vi "Shutdown.vi"(8 "error in":errorcluster, 11 "tCRD in":refnum<class "Open Path CRD.lvclass">) -> (0 "error out":errorcluster, 3 "tCRD out":refnum<class "Open Path CRD.lvclass">)   [LabVIEW 2015, in "Open Path CRD.lvclass"]
uses:
  Open Path CRD.lvclass
  Reusable/Session APIs/File Access/Base/File Session.lvclass
  Open Path CRD.lvclass/Open Path CRD.ctl
  <vilib>/FPGAPlugInAG/sbRIO-9637/niLvFpga_Close_sbRIO-9637.vi
  Reusable/CRDS/Main/CRDS.lvclass
  <vilib>/rvi/interface/nirviCloseFPGA/nirviCloseFPGA.xnode
  Open Path FPGA Ref.ctl
  FPGA Bitfiles/80MHz_server.lvbitx
  Devices/Alicat/Session Based/Alicat Device.lvclass
  Devices/CR5/CR5.lvclass
  <userlib>/_Session Fwk/Session - Root.lvclass
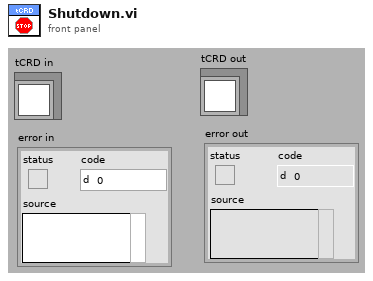
[diagram p1: front panel]
types:
  T1 = typedef "Open Path CRD.lvclass/Open Path FPGA Ref.ctl" = refnum<k20>
  T2 = typedef "Config Data.lvclass/Config Session.ctl" = refnum<data-value>
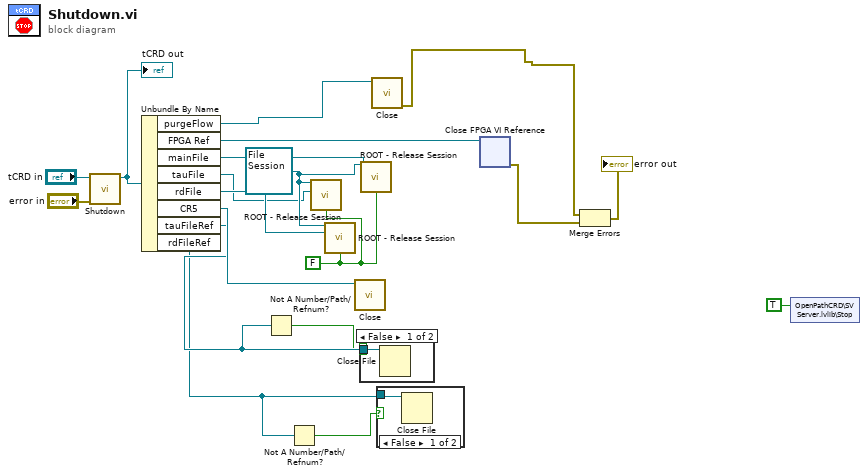
[diagram p0: block diagram]
diagram:
  w6 = FALSE ("force destroy? (F)")
  w10 = refnum<class "File Session.lvclass"> refnum ("File Session")
  n1 = call-parent "Shutdown.vi"("error in"="error in", "Instrument in"="tCRD in") -> ("Instrument out"=w17:refnum<class "Open Path CRD.lvclass">)  [unwired: 8 in, 1 out]
  "tCRD out" <- w17
  n2 = Unbundle By Name(w17) -> ("purgeFlow"=w13:refnum<class "Alicat Device.lvclass">, "FPGA Ref"=w16:T1, "mainFile"=w7:T2, "tauFile"=w8:T2, "rdFile"=w9:T2, "CR5"=w11:refnum<class "CR5.lvclass">, "tauFileRef"=w4:refnum<file>, "rdFileRef"=w3:refnum<file>)
  n3 = Not A Number/Path/Refnum?(number/path/refnum=w4) -> (NaN/Path/Refnum?=w1:bool)
  n4 = Not A Number/Path/Refnum?(number/path/refnum=w3) -> (NaN/Path/Refnum?=w2:bool)
  n5 = call <userlib>:"ROOT - Release Session.vi"("OBJ - Session in"=w10, "Session Handle in"=w8, "force destroy? (F)"=w6) -> ()  [unwired: 11 in, 2 out]
  n6 = call <userlib>:"ROOT - Release Session.vi"("OBJ - Session in"=w10, "Session Handle in"=w9, "force destroy? (F)"=w6) -> ()  [unwired: 11 in, 2 out]
  n7 = call-dynamic "Close.vi"("CR5 in"=w11) -> ()  [unwired: 9 in, 2 out]
  n8 = case shown="False" w1 {
    tunnel: w4 -> [w20 _]
    frame False {
      n9 = Close File(refnum=w20) -> ()  [unwired: 1 in, 2 out]
    }
    frame True {
    }
  }
  n10 = call <userlib>:"ROOT - Release Session.vi"("OBJ - Session in"=w10, "Session Handle in"=w7, "force destroy? (F)"=w6) -> ()  [unwired: 11 in, 2 out]
  n11 = call-dynamic "Close.vi"("Cfg Dev in"=w13) -> ("error out"=w12:errorcluster)  [unwired: 9 in, 1 out]
  n12 = case shown="False" w2 {
    tunnel: w3 -> [w21 _]
    frame False {
      n13 = Close File(refnum=w21) -> ()  [unwired: 1 in, 2 out]
    }
    frame True {
    }
  }
  n14 = xnode "Close FPGA VI Reference"("FPGA VI Reference In"=w16) -> ("error out"=w15:errorcluster)  [unwired: 1 in]
  n15 = Merge Errors(w12, w15) -> (→"error out":errorcluster)
  n16 = shared-variable "OpenPathCRD\\SV Server.lvlib\\Stop"(TRUE ("Stop")) -> ()  [unwired: 1 in, 1 out]
